vi "Target Logging Array Manager.vi"(7 "Allocate New Array":bool, 8 "Input Array":dbl[][](array[numeric]), 9 "Number of Data Columns":i32, 11 "Previous Index":i32) -> (0 "Output Array":dbl[][](array[numeric]), 3 "Array Index to Write":i32)   [LabVIEW 2018]
panel:
  out "Real Time Loop Period Time [microsec]":u32
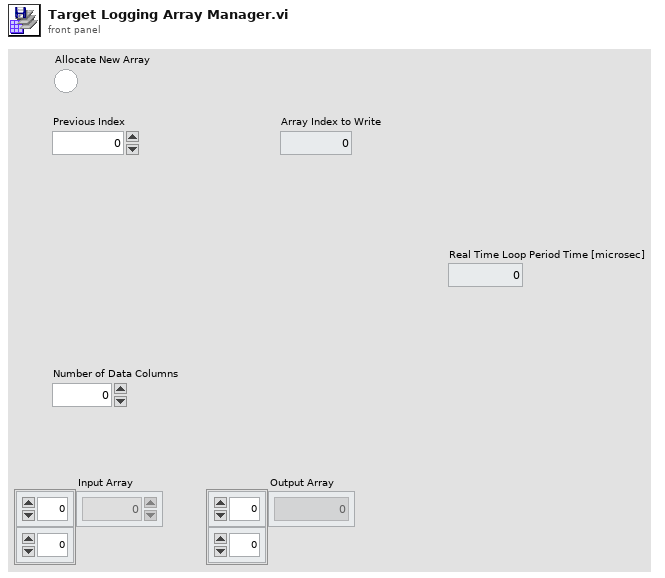
[diagram p1: front panel]
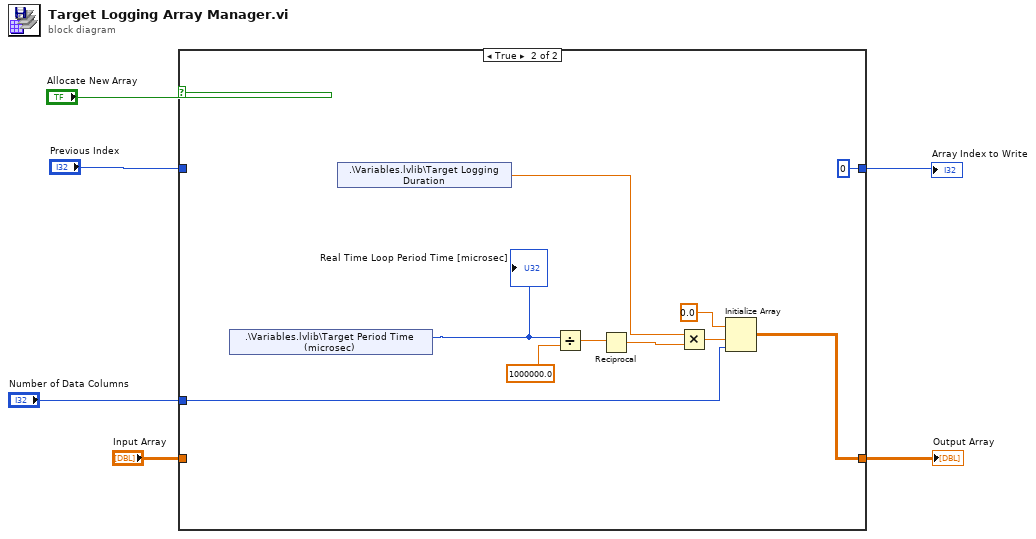
[diagram p0: block diagram]
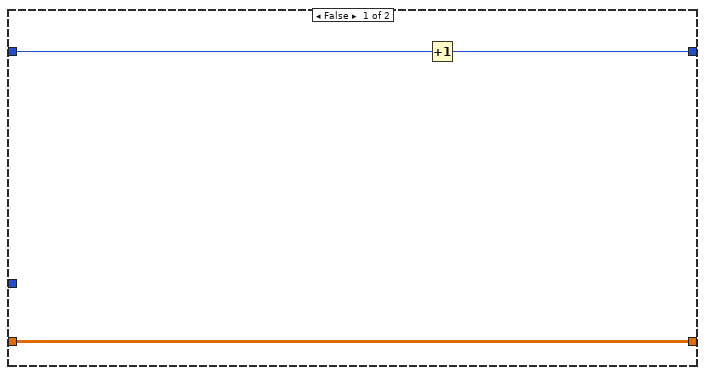
[diagram p2: hidden frame]
diagram:
  n1 = case shown="True" "Allocate New Array" {
    tunnel: "Number of Data Columns" -> [_ w12]
    tunnel: "Input Array" -> [w7 _]
    tunnel: [w7 w14] -> w2
    tunnel: [w9 0] -> w5
    tunnel: "Previous Index" -> [w8 _]
    frame False {
      n2 = Increment(x=w8) -> (x+1=w9:i32)
    }
    frame True {
      n3 = shared-variable ".\\Variables.lvlib\\Target Period Time (microsec)"() -> (w10:u16)  [unwired: 1 in, 1 out]
      "Real Time Loop Period Time [microsec]" <- w10
      n4 = shared-variable ".\\Variables.lvlib\\Target Logging Duration"() -> (w11:dbl)  [unwired: 1 in, 1 out]
      n5 = Divide(x=w10, y=1000000.0) -> (x/y=w16:dbl)
      n6 = Reciprocal(x=w16) -> (1/x=w15:dbl)
      n7 = Multiply(x=w11, y=w15) -> (x*y=w18:dbl)
      n8 = Initialize Array "Initialize Array"(0.0 ("element"), w18, w12) -> (w14:dbl[][])
    }
  }
  "Array Index to Write" <- w5
  "Output Array" <- w2
